vi "AB_User_Log_Start_Time.vi"(7 "action":enum16{"get", "set"}(ring), 8 "error in (no error)":errorcluster) -> (0 "error out":errorcluster, 1 "start time":timestamp)   [LabVIEW 2020]
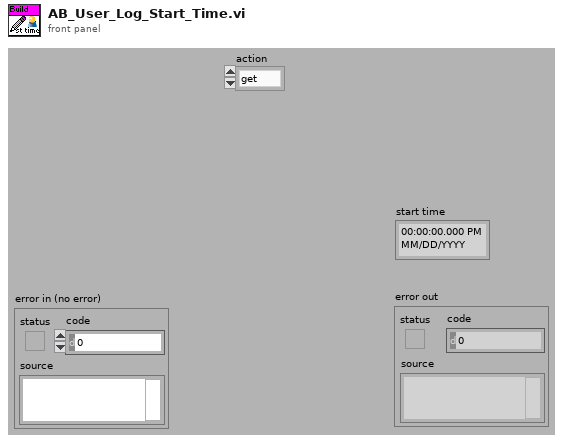
[diagram p1: front panel]
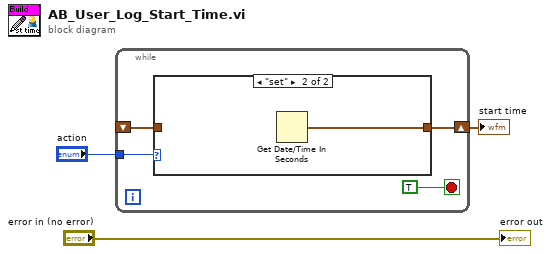
[diagram p0: block diagram]
diagram:
  n1 = while {
    tunnel: "action" -> [w6]
    shift-right: [w5] -> w1
    shift-left: _ -> [w4]
    stop <- TRUE stop-if-true
    n2 = case shown="\"set\"" w6 {
      tunnel: [w8 w9] -> w5
      tunnel: w4 -> [w8 _]
      frame "get" {
      }
      frame "set" {
        n3 = Get Date/Time In Seconds() -> (seconds since 1Jan1904=w9:timestamp)
      }
    }
  }
  "start time" <- w1
  "error out" <- "error in (no error)"
